vi "No_Name_Size.vi"() -> (0 "数组":string[][](array[string]))   [LabVIEW 2011]
panel:
  # "将HASS 协议中的数据格式_名称_内存大小 \n以数组常量的格式存储方便搜索用"
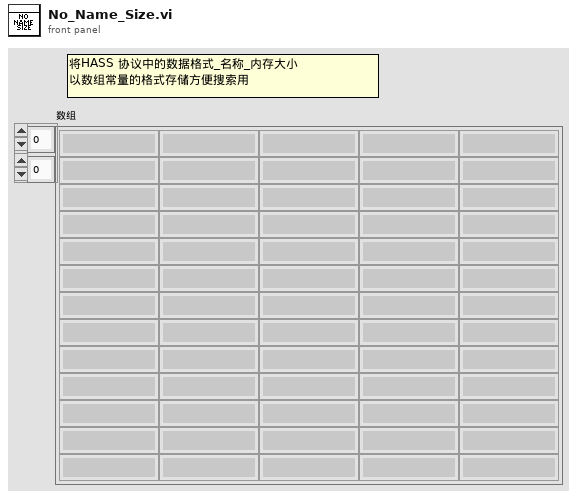
[diagram p1: front panel]
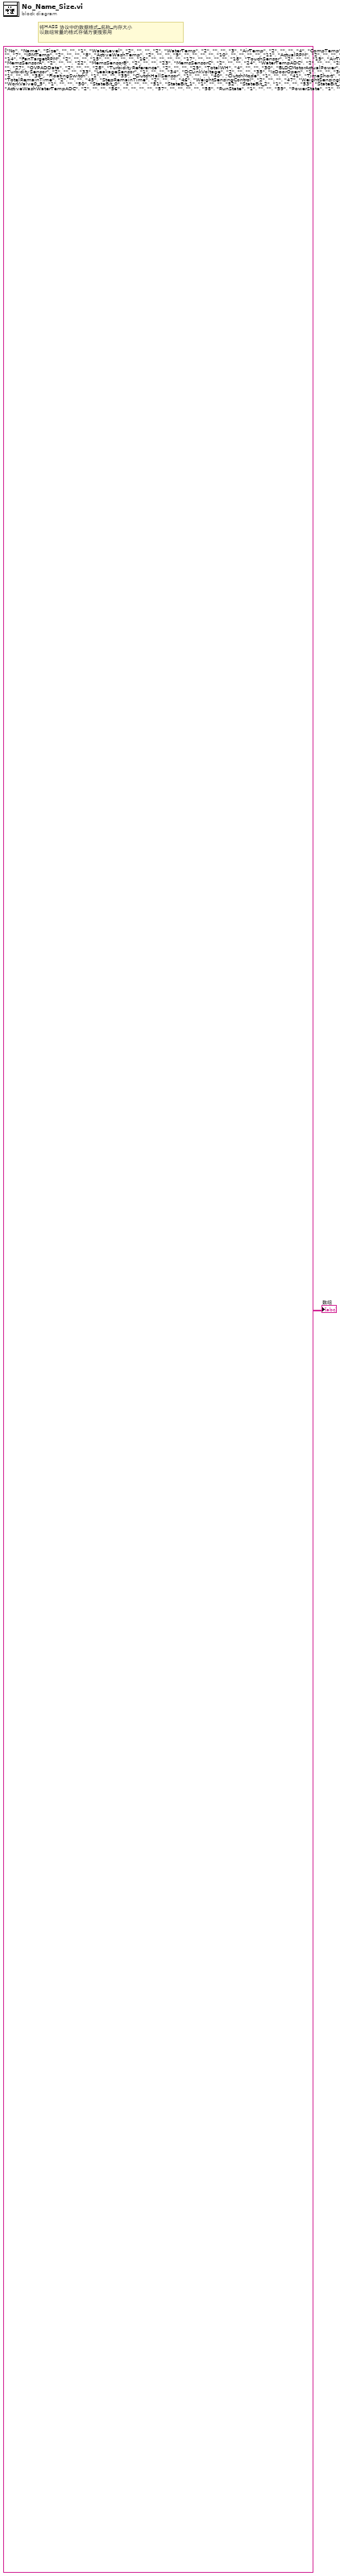
[diagram p0: block diagram]
diagram:
  # "将HASS 协议中的数据格式_名称_内存大小 \n以数组常量的格式存储方便搜索用"
  "数组" <- string[][] [["No", "Name", "Size", "", ""], ["1", "WaterLevel", "2", "", ""], ["2", "WaterTemp", "2", "", ""], ["3", "AirTemp", "2", "", ""], ["4", "CompTemp", "2", "", ""], ["5", "FilterTemp", "2", "", ""], ["6", "VentTemp", "2", "", ""], ["7", "IPMTemp", "2", "", ""], ["8", "ActiveWashTemp", "2", "", ""], ["9", "", "", "", ""], ["10", "", "", "", ""], ["11", "ActualRPM", "2", "", ""], ["12", "TargettingRPM", "2", "", ""], ["13", "FanActualRPM", "2", "", ""], ["14", "FanTargetRPM", "2", "", ""], ["15", "", "", "", ""], ["16", "", "", "", ""], ["17", "", "", "", ""], ["18", "TouchSensor", "2", "", ""], ["19", "AirTermistorADC", "2", "", ""], ["20", "VentTermistorADC", "2", "", ""], ["21", "MemsSensorA", "2", "", ""], ["22", "MemsSensorB", "2", "", ""], ["23", "MemsSensorC", "2", "", ""], ["24", "WaterTempADC", "2", "", ""], ["25", "OverflowADData", "2", "", ""], ["26", "LeakageADData", "2", "", ""], ["27", "OVPADData", "2", "", ""], ["28", "TurbidityReference", "2", "", ""], ["29", "TotalWH", "4", "", ""], ["30", "BLDCMotorActualPower", "2", "", ""], ["31", "TouchSensor", "2", "", ""], ["32", "TurbiditySensor", "2", "", ""], ["33", "LeakageSensor", "1", "", ""], ["34", "DCLinkVoltage", "2", "", ""], ["35", "IsDoorOpen", "1", "", ""], ["36", "AutoDispensorOpenDetect", "1", "", ""], ["37", "CheckerSwitch", "1", "", ""], ["38", "FloatingSwitch", "1", "", ""], ["39", "ClutchHallSensor", "1", "", ""], ["40", "ClutchMode", "1", "", ""], ["41", "TimeShort", "1", "", ""], ["42", "Progress", "1", "", ""], ["43", "Step", "1", "", ""], ["44", "TotalRemainTime", "2", "", ""], ["45", "StepRemainTime", "2", "", ""], ["46", "WeightSensingControl", "2", "", ""], ["47", "WeightSensingResult", "1", "", ""], ["48", "WaterValve0_7", "1", "", ""], ["49", "WorkValve0_5", "1", "", ""], ["50", "StateBit_0", "1", "", ""], ["51", "StateBit_1", "1", "", ""], ["52", "StateBit_2", "1", "", ""], ["53", "StateBit_3", "1", "", ""], ["54", "StateBit_4", "1", "", ""], ["55", "ActiveWashWaterTempADC", "2", "", ""], ["56", "", "", "", ""], ["57", "", "", "", ""], ["58", "RunState", "1", "", ""], ["59", "PowerState", "1", "", ""], ["60", "SoundID", "1", "", ""], ["61", "ErrorCode", "4", "", ""], ["62", "TotalFlowMeterPulse", "2", "", ""], ["63", "FlowMeterPulse", "2", "", ""], ["64", "WaterSoftnerRegenSettingLevel", "1", "", ""], ["65", "RinseAidShortage", "1", "", ""], ["66", "WaterSoftnerSaltShortage", "1", "", ""], ["67", "LowWaterLevelSwitchSensed", "1", "", ""], ["68", "SensedIVTDoorOpened", "1", "", ""], ["69", "SensedMotorErrorFromIVT", "1", "", ""], ["70", "LowLevelSensingReferencePower", "2", "", ""], ["71", "DistributorPosition", "1", "", ""], ["72", "DistributorSWSensingSignal ", "1", "", ""], ["73", "VaneResetSignal", "1", "", ""], ["74", "SensedTurbidityLevel", "1", "", ""], ["75", "", "", "", ""], ["76", "IVTCtrlResponseType", "1", "", ""], ["77", "IsDoorLocked", "1", "", ""], ["78", "MotorOnTime", "2", "", ""], ["79", "MotorOffTime", "2", "", ""], ["80", "SudsDetect", "2", "", ""], ["81", "OverloadDetect", "2", "", ""], ["82", "OptionData", "2", "", ""], ["83", "CourseRecipeData", "15", "", ""], ["84", "DryerStateBit0_7", "1", "", ""], ["85", "", "", "", ""], ["86", "", "", "", ""], ["87", "", "", "", ""], ["88", "", "", "", ""], ["89", "", "", "", ""], ["90", "", "", "", ""], ["91", "", "", "", ""], ["92", "", "", "", ""], ["93", "", "", "", ""], ["94", "", "", "", ""], ["95", "", "", "", ""], ["96", "", "", "", ""], ["97", "", "", "", ""], ["98", "", "", "", ""], ["99", "", "", "", ""], ["100", "", "", "", ""], ["101", "KeyData1", "4", "", ""], ["102", "KeyData2", "4", "", ""], ["103", "PowerKey", "1", "", ""], ["104", "KeyPushTime", "4", "", ""], ["105", "", "", "", ""], ["106", "", "", "", ""], ["107", "", "", "", ""], ["108", "", "", "", ""], ["109", "", "", "", ""], ["110", "", "", "", ""], ["111", "", "", "", ""], ["112", "", "", "", ""], ["113", "", "", "", ""], ["114", "", "", "", ""], ["115", "", "", "", ""], ["116", "", "", "", ""], ["117", "", "", "", ""], ["118", "", "", "", ""], ["119", "", "", "", ""], ["120", "", "", "", ""], ["121", "", "", "", ""], ["122", "", "", "", ""], ["123", "", "", "", ""], ["124", "", "", "", ""], ["125", "", "", "", ""], ["126", "", "", "", ""], ["127", "", "", "", ""], ["128", "", "", "", ""], ["129", "", "", "", ""], ["130", "", "", "", ""], ["131", "", "", "", ""], ["132", "", "", "", ""], ["133", "", "", "", ""], ["134", "", "", "", ""], ["135", "", "", "", ""], ["136", "", "", "", ""], ["137", "", "", "", ""], ["138", "", "", "", ""], ["139", "", "", "", ""], ["140", "", "", "", ""], ["141", "", "", "", ""], ["142", "", "", "", ""], ["143", "", "", "", ""], ["144", "", "", "", ""], ["145", "", "", "", ""], ["146", "", "", "", ""], ["147", "", "", "", ""], ["148", "", "", "", ""], ["149", "", "", "", ""], ["150", "", "", "", ""], ["151", "UTADATA1", "30", "", ""], ["152", "UTADATA2", "30", "", ""], ["153", "UTADATA3", "30", "", ""], ["154", "", "", "", ""], ["155", "", "", "", ""], ["156", "", "", "", ""], ["157", "", "", "", ""], ["158", "", "", "", ""], ["159", "RecentCourse1st", "5", "", ""], ["160", "RecentCourse2nd", "5", "", ""], ["161", "RecentCourse3rd", "5", "", ""], ["162", "RecentCourse4th", "5", "", ""], ["163", "RecentCourse5th", "5", "", ""], ["164", "", "", "", ""], ["165", "", "", "", ""], ["166", "", "", "", ""], ["167", "", "", "", ""], ["168", "", "", "", ""], ["169", "", "", "", ""], ["170", "", "", "", ""], ["171", "", "", "", ""], ["172", "", "", "", ""], ["173", "", "", "", ""], ["174", "", "", "", ""], ["175", "", "", "", ""], ["176", "", "", "", ""], ["177", "", "", "", ""], ["178", "", "", "", ""], ["179", "", "", "", ""], ["180", "", "", "", ""], ["181", "", "", "", ""], ["182", "", "", "", ""], ["183", "", "", "", ""], ["184", "", "", "", ""], ["185", "", "", "", ""], ["186", "", "", "", ""], ["187", "", "", "", ""], ["188", "", "", "", ""], ["189", "", "", "", ""], ["190", "", "", "", ""], ["191", "", "", "", ""], ["192", "", "", "", ""], ["193", "", "", "", ""], ["194", "", "", "", ""], ["195", "", "", "", ""], ["196", "", "", "", ""], ["197", "", "", "", ""], ["198", "", "", "", ""], ["199", "", "", "", ""], ["200", "", "", "", ""], ["201", "VersionMain", "4", "", ""], ["202", "VersionSub", "4", "", ""], ["203", "VersionInverter", "4", "", ""], ["204", "VersionTocuh", "4", "", ""], ["205", "VersionLCD", "4", "", ""], ["206", "VersionWiFi", "4", "", ""], ["207", "VersionEEPROMImage", "4", "", ""], ["208", "", "", "", ""], ["209", "", "", "", ""], ["210", "", "", "", ""], ["211", "", "", "", ""], ["212", "", "", "", ""], ["213", "", "", "", ""], ["214", "", "", "", ""], ["215", "", "", "", ""], ["216", "", "", "", ""], ["217", "", "", "", ""], ["218", "", "", "", ""], ["219", "", "", "", ""], ["220", "RecentErrorData", "5", "", ""], ["221", "", "", "", ""], ["222", "", "", "", ""], ["223", "", "", "", ""], ["224", "", "", "", ""], ["225", "", "", "", ""], ["226", "HASS", "1", "", ""], ["227", "SmartInstallIndex", "1", "", ""], ["228", "SmartInstallState", "1", "", ""], ["229", "TestMode", "2", "", ""], ["230", "SerialNumber", "15", "", ""], ["231", "InLineWriting", "22", "", ""], ["232", "ProductType", "1", "", ""], ["233", "InLineWritingSuccess", "1", "", ""], ["234", "", "", "", ""], ["235", "", "", "", ""], ["236", "", "", "", ""], ["237", "", "", "", ""], ["238", "", "", "", ""], ["239", "", "", "", ""], ["240", "", "", "", ""], ["241", "", "", "", ""], ["242", "", "", "", ""], ["243", "", "", "", ""], ["244", "", "", "", ""], ["245", "", "", "", ""], ["246", "", "", "", ""], ["247", "", "", "", ""], ["248", "", "", "", ""], ["249", "", "", "", ""], ["250", "", "", "", ""], ["251", "RequestDataToTarget", "1", "", ""], ["252", "", "", "", ""], ["253", "", "", "", ""], ["254", "", "", "", ""], ["255", "", "", "", ""]]
